vi "Init Events.vi"(8 "error in (no error)":errorcluster, 11 "AppDetailPanel in":refnum<class "AppDetailPanel.lvclass">) -> (0 "error out":errorcluster, 3 "AppDetailPanel out":refnum<class "AppDetailPanel.lvclass">)   [LabVIEW 2020, in "PicoG-App.lvlib" / "AppDetailPanel.lvclass"]
uses:
  AppDetailPanel.lvclass
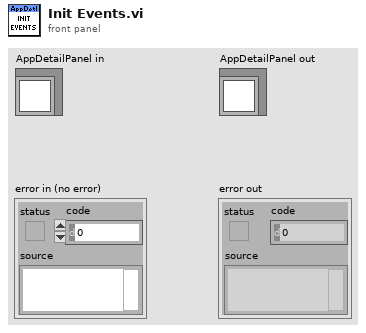
[diagram p1: front panel]
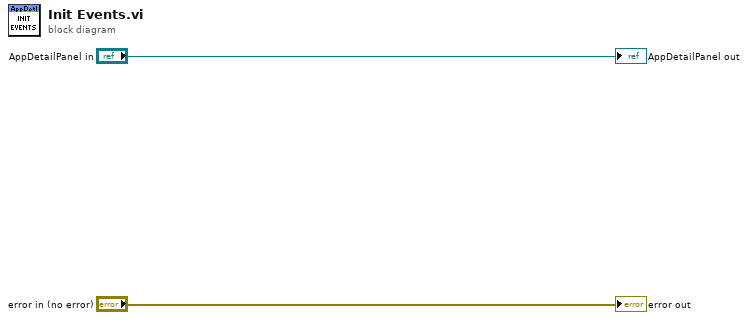
[diagram p0: block diagram]
diagram:
  "error out" <- "error in (no error)"
  "AppDetailPanel out" <- "AppDetailPanel in"
